vi "Write Project controls refs.vi"(8 "error in (no error)":errorcluster, 10 "Def_DB_FP_commands":T1, 11 "DB in":refnum<class "DB.lvclass">) -> (0 "error out":errorcluster, 3 "DB out":refnum<class "DB.lvclass">)   [LabVIEW 2015, in "DB.lvclass"]
uses:
  DB.lvclass
  Def_DB_FP_ref_commands.ctl
  DB.lvclass/DB.ctl
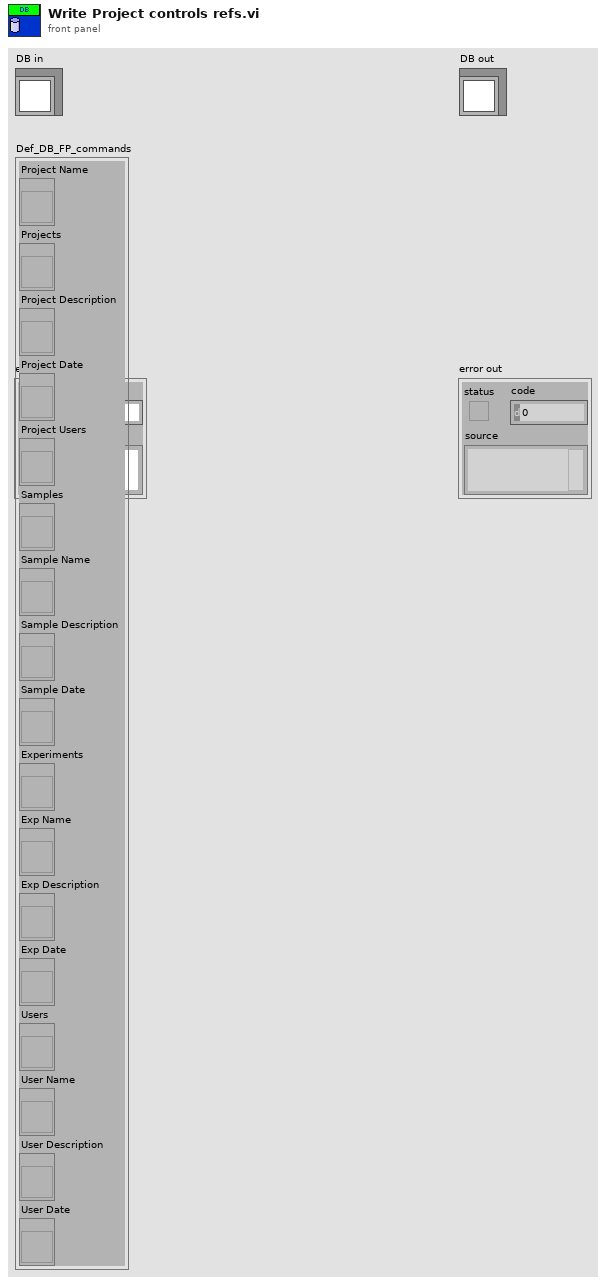
[diagram p1: front panel]
types:
  T1 = typedef "Def_DB_FP_ref_commands.ctl" = cluster{"Project Name":refnum<vi>, "Projects":refnum<vi>, "Project Description":refnum<vi>, "Project Date":refnum<vi>, "Project Users":refnum<vi>, "Samples":refnum<vi>, "Sample Name":refnum<vi>, "Sample Description":refnum<vi>, "Sample Date":refnum<vi>, "Experiments":refnum<vi>, "Exp Name":refnum<vi>, "Exp Description":refnum<vi>, "Exp Date":refnum<vi>, "Users":refnum<vi>, "User Name":refnum<vi>, "User Description":refnum<vi>, "User Date":refnum<vi>}
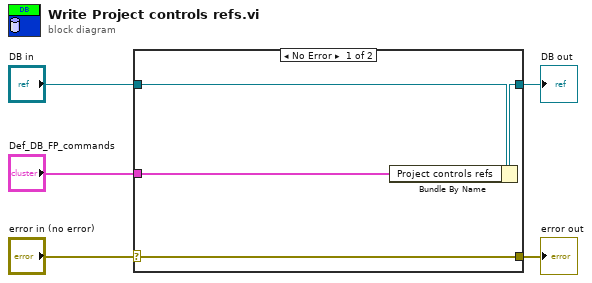
[diagram p0: block diagram]
diagram:
  n1 = case shown="No Error" "error in (no error)" {
    selector: "error in (no error)" -> [w9 w10]
    tunnel: [w9 w10] -> w4
    tunnel: [w7 w11] -> w2
    tunnel: "DB in" -> [w8 w11]
    tunnel: "Def_DB_FP_commands" -> [w6 _]
    frame No Error {
      n2 = Bundle By Name(cluster=w8, "Project controls refs"=w6) -> (w7:refnum<class "DB.lvclass">)
    }
    frame Error {
    }
  }
  "error out" <- w4
  "DB out" <- w2
